vi "crosshairs.vi"(9 "y":dbl=497.0 format="%#_13g", 10 "x":dbl=400.0 format="%#_13g", 11 "Refnum in":T1) -> (3 "Refnum out":T1)   [LabVIEW 2015]
uses:
  <vilib>/vision/Image Controls.llb/IMAQ Image.ctl
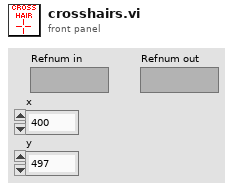
[diagram p1: front panel]
types:
  T1 = typedef "IMAQ Image.ctl" = refnum<image>
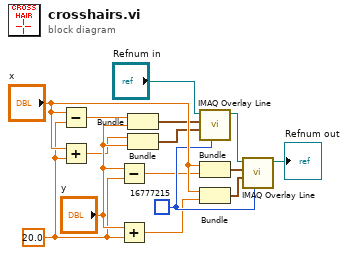
[diagram p0: block diagram]
diagram:
  w11 = u32 16777215 ("Color")
  w6 = 20.0
  n1 = Subtract(x="x", y=w6) -> (x-y=w2:dbl)
  n2 = Add(x="x", y=w6) -> (x+y=w4:dbl)
  n3 = Subtract(x="y", y=w6) -> (x-y=w7:dbl)
  n4 = Add(x="y", y=w6) -> (x+y=w8:dbl)
  n5 = Bundle(w2, "y"="y") -> (w3:cluster{dbl, "y":dbl})  [unwired: 1 in]
  n6 = Bundle(w4, "y"="y") -> (w5:cluster{dbl, "y":dbl})  [unwired: 1 in]
  n7 = call "IMAQ Overlay Line"("Color"=w11, "End Point"=w5, "Start Point"=w3, "Image"="Refnum in") -> ("Image Out"=w12:T1)  [unwired: 6 in, 1 out]
  n8 = Bundle("x"="x", w7) -> (w9:cluster{"x":dbl, dbl})  [unwired: 1 in]
  n9 = Bundle("x"="x", w8) -> (w10:cluster{"x":dbl, dbl})  [unwired: 1 in]
  n10 = call "IMAQ Overlay Line"("Color"=w11, "End Point"=w10, "Start Point"=w9, "Image"=w12) -> ("Image Out"=→"Refnum out":T1)  [unwired: 6 in, 1 out]
